vi "Move Active Pixels Down.vi"(8 "error in (no error)":errorcluster, 10 "Boolean":bool, 11 "Game Engine in":refnum<class "Game Engine.lvclass">) -> (0 "error out":errorcluster, 3 "Game Engine out":refnum<class "Game Engine.lvclass">)   [LabVIEW 2017, in "Game Engine.lvlib" / "Game Engine.lvclass"]
uses:
  Game Engine.lvclass
  Game Engine.lvclass/Game Engine.ctl
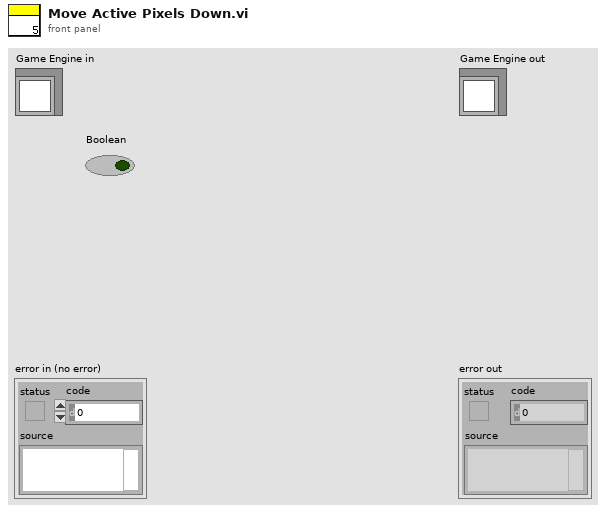
[diagram p1: front panel]
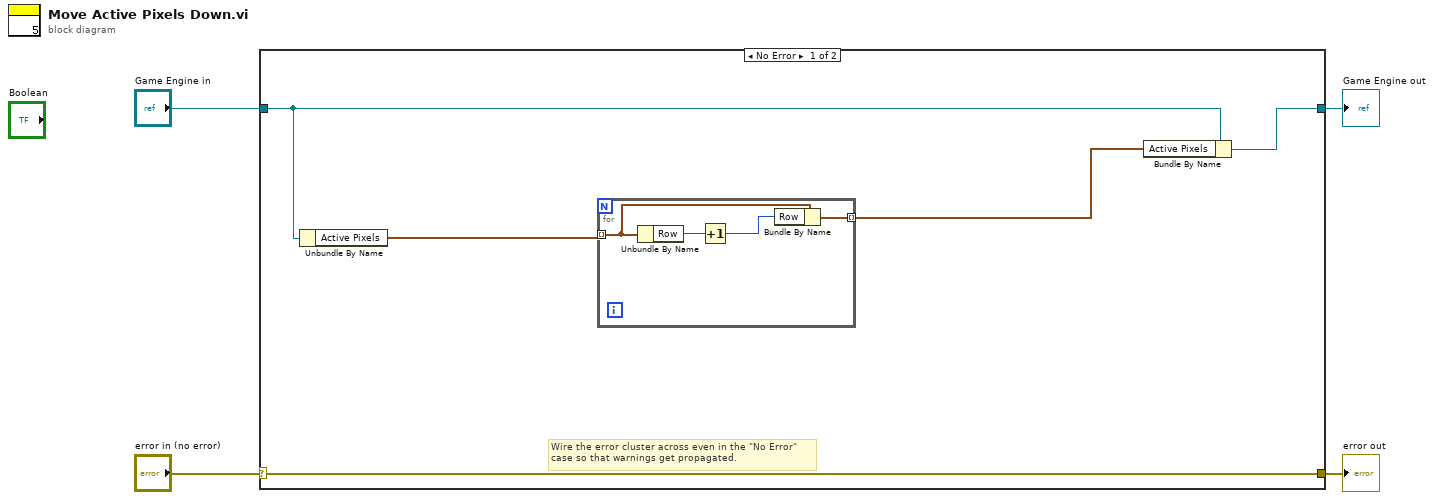
[diagram p0: block diagram]
diagram:
  n1 = case shown="No Error" "error in (no error)" {
    selector: "error in (no error)" -> [w9 w15]
    tunnel: [w9 w15] -> w3
    tunnel: [w6 w14] -> w1
    tunnel: "Game Engine in" -> [w7 w14]
    frame No Error {
      # "Wire the error cluster across even in the \"No Error\"\ncase so that warnings get propagated."
      n2 = Unbundle By Name(w7) -> ("Active Pixels"=w8:cluster{"Column":u8, "Row":u8, "Color":u32}[])
      n3 = for {
        tunnel: w8 -> [w12] mode=indexing
        tunnel: [w10] -> w5 mode=indexing
        n4 = Unbundle By Name(w12) -> ("Row"=w13:u8)
        n5 = Increment(x=w13) -> (x+1=w11:u8)
        n6 = Bundle By Name(cluster=w12, "Row"=w11) -> (w10:cluster{"Column":u8, "Row":u8, "Color":u32})
      }
      n7 = Bundle By Name(cluster=w7, "Active Pixels"=w5) -> (w6:refnum<class "Game Engine.lvclass">)
    }
    frame Error {
    }
  }
  "error out" <- w3
  "Game Engine out" <- w1
